vi "Choreo_TrajectoryState_GetTime.vi"(11 "ChoreoTrajectoryState":T1) -> (3 "timestamp":dbl)   [LabVIEW 2019, in "ChoreoLib.lvlib"]
doc: "Return the timestamp of this state. This is the elapsed seconds from the start of the trajectory.\n\nInputs:\n - ChoreoTrajectoryState - cluster - Individual trajectory state\n\nOutputs: \n - timestamp - double - The timestamp of this state. Seconds."
uses:
  ChoreoLib.lvlib
  TypeDef/ChoreoTrajectoryState.ctl
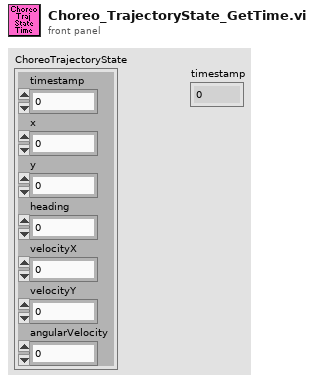
[diagram p1: front panel]
types:
  T1 = typedef "ChoreoLib.lvlib/ChoreoTrajectoryState.ctl" = cluster{"timestamp":dbl, "x":dbl, "y":dbl, "heading":dbl, "velocityX":dbl, "velocityY":dbl, "angularVelocity":dbl}
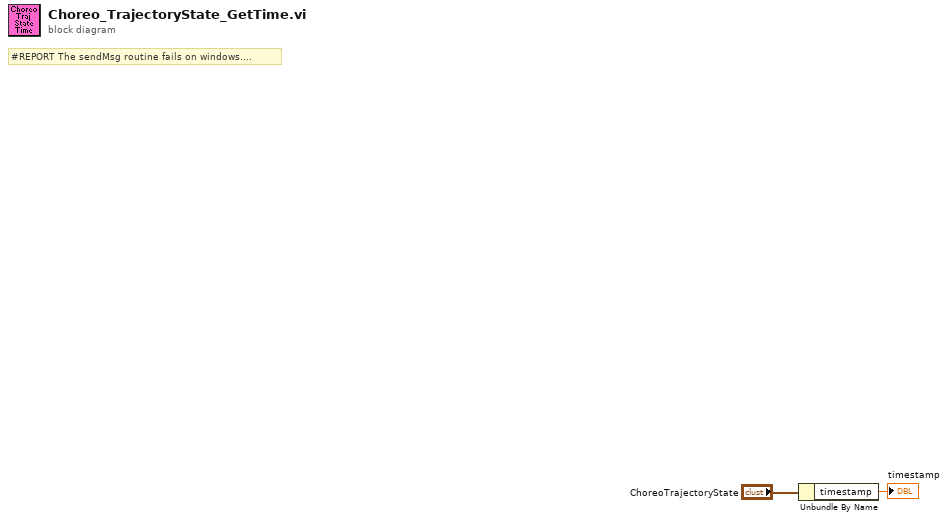
[diagram p0: block diagram]
diagram:
  # "#REPORT The sendMsg routine fails on windows...."
  n1 = Unbundle By Name("ChoreoTrajectoryState") -> ("timestamp"=→"timestamp":dbl)
